vi "Write Data.vi"(10 "Data":cluster{"EDR":dbl, "Pulse":u8}, 11 "Data Update Msg in":refnum<class "Data Update Msg.lvclass">) -> (3 "Data Update Msg out":refnum<class "Data Update Msg.lvclass">)   [LabVIEW 2011, in "Data Update Msg.lvclass"]
uses:
  Data Update Msg.lvclass
  Data Update Msg.lvclass/Data Update Msg.ctl
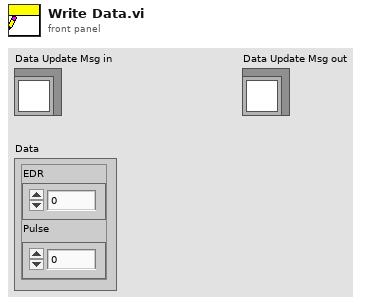
[diagram p1: front panel]
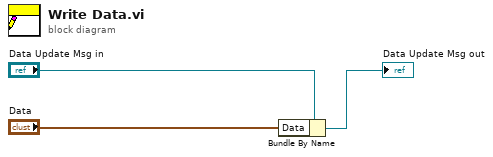
[diagram p0: block diagram]
diagram:
  n1 = Bundle By Name(cluster="Data Update Msg in", "Data"="Data") -> (→"Data Update Msg out":refnum<class "Data Update Msg.lvclass">)
